vi "Vision_Processing_L_R1.vi"(0 "Current State":enum16{"Short Range", "Long Range"}(ring)=enum."Long Range", 1 "Image Dst":T1=refnum, 2 "Inpute Image":T1=refnum, 3 "Startup Flag":bool, 4 "Valid Beacon History - in":bool[](array[boolean])=[TRUE, TRUE, TRUE, TRUE, TRUE, TRUE, TRUE, TRUE, TRUE, TRUE, TRUE, TRUE, TRUE, TRUE, TRUE, TRUE, TRUE, TRUE, TRUE, TRUE], 5 "Current ROI Descriptor":T7={"Global Rectangle"=[0, 126, 320, 179], "Contours"=[{"ID"=enum."External", "Type"=12, "Coordinates"=[0, 126, 320, 179, 0]}]} {"Contours"."Type" items=["No Selection", "Point", "Line", "Rectangle", "Oval", "Polygon", "Freehand Region", "Annulus", "Unused2", "Unused3", "Broken Line", "Freehand Line", "Rotated Rectangle"]}, 6 "Avg Score - Last":dbl=882.2747192382812, 7 "error in (no error)":errorcluster, 8 "Current Settings":T4={"Curve Parameters"={"Extraction Mode"=1, "Edge Threshold"=150, "Edge Filter Size"=0, "Min Length"=25, "Row Search Step Size"=15, "Col Search Step Size"=15, "Max Endpoint Gap"=2, "Closed"=TRUE, "Subpixel"=TRUE}, "Match Mode"={"Rotation"=TRUE, "Scale"=TRUE, "Occlusion"=TRUE, "Reserved"=FALSE, "Reserved"=FALSE, "Reserved"=FALSE}, "Range Settings"=[{"Match Constraints"=0, "Min"=-5.0, "Max"=5.0}, {"Match Constraints"=1, "Min"=77.28628845214844, "Max"=87.28628845214844}, {"Match Constraints"=2, "Min"=0.0, "Max"=25.0}], "Number of Matches"=1, "Minimum Match Score"=782.2747, "SubPixel Accuracy"=TRUE, "Adv. Geometric Match Options 2"=[{"Setup Data Item"=20, "Item Value"=0.0}, {"Setup Data Item"=22, "Item Value"=1.0}]} {"Curve Parameters"."Extraction Mode" items=["Normal", "Uniform Regions"]; "Curve Parameters"."Edge Filter Size" items=["Fine", "Normal", "Contour Tracing"]; "Curve Parameters"."Max Endpoint Gap" min=0; "Curve Parameters"."Col Search Step Size" min=1 max=255 step=1; "Curve Parameters"."Row Search Step Size" min=1 max=255 step=1; "Curve Parameters"."Min Length" min=0; "Curve Parameters"."Edge Threshold" min=1 max=350 step=1; "Range Settings"."Max" format="%.2f"; "Range Settings"."Min" format="%.2f"; "Range Settings"."Match Constraints" items=["Rotation Angle (degrees)", "Scale Factor (%)", "Occlusion (%)"]; "Adv. Geometric Match Options 2"."Setup Data Item" items=["Curve Extraction Mode", "Curve Edge Threshold", "Curve Edge Filter Size", "Min Curve Length", "Curve Row Search Step Size", "Curve Col Search Step Size", "Curve Max Endpoint Gap", "Extract Closed Curves", "Enable Subpixel Curve Extraction", "Enable Correlation Score", "Enable Subpixel Accuracy", "Subpixel Iterations", "Subpixel Tolerance", "Initial Match List Length", "Enable Target Template Curve Score", "Min Match Separation Distance", "Min Match Separation Angle", "Min Match Separation Scale", "Max Match Overlap", "Enable Coarse Result", "Enable Calibration Support", "Enable Contrast Reversal", "Search Strategy", "Refinement Match Factor", "Subpixel Match Factor"]}, 9 "Sub Beacon Search Enable":bool[](array[boolean])=[FALSE, FALSE, FALSE, FALSE, FALSE], 13 "Avg Scale - Last":dbl=82.28628845214844, 14 "Valid Score History":dbl[](array[numeric])=[882.2267456054688, 879.6480102539062, 889.1240844726562, 884.991455078125, 875.38330078125, 881.3228759765625, 879.0923461914062, 884.8130493164062, 869.0428466796875, 879.3259887695312, 878.3837280273438, 878.5771484375, 878.74462890625, 883.9327392578125, 889.0577392578125, 886.224365234375, 888.1887817382812, 886.6435546875, 888.8932495117188, 880.26025390625] format="%#_13g", 15 "Valid Scale History":dbl[](array[numeric])=[86.3126220703125, 81.15679931640625, 81.2668228149414, 81.51744842529297, 81.17774963378906, 81.44428253173828, 81.47639465332031, 81.52884674072266, 81.38125610351562, 86.32369232177734, 81.46265411376953, 81.3922348022461, 81.34772491455078, 81.08159637451172, 81.33423614501953, 81.38683319091797, 81.22872924804688, 81.17185974121094, 81.34151458740234, 81.41799926757812] format="%#_13g", 16 "History Size":i32=20) -> (10 "Valid Scale History\nOut":dbl[](array[numeric])=[81.32903289794922, 86.3126220703125, 81.15679931640625, 81.2668228149414, 81.51744842529297, 81.17774963378906, 81.44428253173828, 81.47639465332031, 81.52884674072266, 81.38125610351562, 86.32369232177734, 81.46265411376953, 81.3922348022461, 81.34772491455078, 81.08159637451172, 81.33423614501953, 81.38683319091797, 81.22872924804688, 81.17185974121094, 81.34151458740234] format="%#_13g", 11 "Avg Scale":dbl=82.31654510498046, 12 "Avg Score":dbl=881.4775024414063, 17 "Valid Score History\nOut":dbl[](array[numeric])=[871.397216796875, 882.2267456054688, 879.6480102539062, 889.1240844726562, 884.991455078125, 875.38330078125, 881.3228759765625, 879.0923461914062, 884.8130493164062, 869.0428466796875, 879.3259887695312, 878.3837280273438, 878.5771484375, 878.74462890625, 883.9327392578125, 889.0577392578125, 886.224365234375, 888.1887817382812, 886.6435546875, 888.8932495117188] format="%#_13g", 18 "Valid Beacon History\nOut":bool[](array[boolean])=[TRUE, TRUE, TRUE, TRUE, TRUE, TRUE, TRUE, TRUE, TRUE, TRUE, TRUE, TRUE, TRUE, TRUE, TRUE, TRUE, TRUE, TRUE, TRUE, TRUE], 19 "Y Coordinates":sgl[](array[numeric])=[0.0, 0.0, 153.47913, 150.49385, 148.50107], 20 "Beacons Found":bool[](array[boolean])=[FALSE, FALSE, TRUE, TRUE, TRUE], 21 "X Coordinates":sgl[](array[numeric])=[0.0, 0.0, 161.30458, 216.11124, 265.1904], 22 "Next Main ROI Descriptor":T6={"Global Rectangle"=[0, 126, 320, 176], "Contours"=[{"ID"=enum."External", "Type"=12, "Coordinates"=[0, 126, 320, 176, 0]}]} {"Contours"."Type" items=["No Selection", "Point", "Line", "Rectangle", "Oval", "Polygon", "Freehand Region", "Annulus", "Unused2", "Unused3", "Broken Line", "Freehand Line", "Rotated Rectangle"]}, 23 "Lock Status":bool=TRUE, 24 "Startup Flag - out":bool, 25 "New Settings":T4={"Curve Parameters"={"Extraction Mode"=1, "Edge Threshold"=150, "Edge Filter Size"=0, "Min Length"=25, "Row Search Step Size"=15, "Col Search Step Size"=15, "Max Endpoint Gap"=2, "Closed"=TRUE, "Subpixel"=TRUE}, "Match Mode"={"Rotation"=TRUE, "Scale"=TRUE, "Occlusion"=TRUE, "Reserved"=FALSE, "Reserved"=FALSE, "Reserved"=FALSE}, "Range Settings"=[{"Match Constraints"=0, "Min"=-5.0, "Max"=5.0}, {"Match Constraints"=1, "Min"=77.31654510498046, "Max"=87.31654510498046}, {"Match Constraints"=2, "Min"=0.0, "Max"=25.0}], "Number of Matches"=1, "Minimum Match Score"=781.4775, "SubPixel Accuracy"=TRUE, "Adv. Geometric Match Options 2"=[{"Setup Data Item"=20, "Item Value"=0.0}, {"Setup Data Item"=22, "Item Value"=1.0}]} {"Curve Parameters"."Extraction Mode" items=["Normal", "Uniform Regions"]; "Curve Parameters"."Edge Filter Size" items=["Fine", "Normal", "Contour Tracing"]; "Curve Parameters"."Max Endpoint Gap" min=0; "Curve Parameters"."Col Search Step Size" min=1 max=255 step=1; "Curve Parameters"."Row Search Step Size" min=1 max=255 step=1; "Curve Parameters"."Min Length" min=0; "Curve Parameters"."Edge Threshold" min=1 max=350 step=1; "Range Settings"."Max" format="%.2f"; "Range Settings"."Min" format="%.2f"; "Range Settings"."Match Constraints" items=["Rotation Angle (degrees)", "Scale Factor (%)", "Occlusion (%)"]}, 26 "Next State":enum16{"Short Range", "Long Range"}(ring)=enum."Long Range", 27 "Right Image 2":T1(plugin-control))   [LabVIEW 2015]
uses:
  <vilib>/vision/Image Controls.llb/IMAQ Image.ctl
  <vilib>/vision/Pattern Matching.llb/IMAQ Curve Parameters.ctl
  <vilib>/vision/Pattern Matching.llb/IMAQ Match Range Setting.ctl
panel:
  in  "Scale Decay \nFactor":dbl=0.5
  in  "Scale Decay \nFactor":dbl=5.0
  in  "Valid Treshold\nfor Lock":i16=5
  in  "Indivudual Beacon \nCushion (pixels)":sgl=5.0
  out "New Min Score":dbl=781.4775024414063
  out "New Low Scale":dbl=77.31654510498046
  out "New high Scale":dbl=87.31654510498046
  in  "Absolute\nMinimum Score":dbl=700.0
  in  "Absolute\nMaximum Scale":dbl=300.0
  in  "Absolute\nMinimum Scale":dbl=10.0
  in  "Default No Lock\nSetting Values":T5={"Min Scale"=50.0, "Max Scale"=150.0, "Min Score"=800.0}
  in  "Score\nCushion":dbl=100.0
  in  "Scale \nCushion":dbl=5.0
  in  "LR to SR\nTransition Scale":sgl=90.0
  in  "SR to LR\nTransition Scale":sgl=90.0
  in  "Timeout \nThrehsold":i32=1000
  in  "Main ROI Decay\nper Fail (pixels)":i32=20
  in  "ROI_factor(Horiztonal) LR":sgl=5.0
  in  "ROI_factor(vertical) LR":sgl=2.5
  in  "ROI_factor(vertical) SR":sgl=2.7
  in  "ROI_factor(Horiztonal) SR":sgl=2.0
  out "Current  Score":sgl=871.3972
  out "Current  Scale":sgl=81.32903
  in  "Fail Count - In":i32
  in  "Sub Beacon Template File Path - ARRAY":path[](array[path])=[path "/home/lvuser/natinst/bin/BeaconTemplates/Sub1.png", path "/home/lvuser/natinst/bin/BeaconTemplates/Sub2.png", path "/home/lvuser/natinst/bin/BeaconTemplates/Sub3.png", path "/home/lvuser/natinst/bin/BeaconTemplates/Sub4.png", path "/home/lvuser/natinst/bin/BeaconTemplates/Sub5.png"]
  in  "Short Range Template FIle Path":path=path "/home/lvuser/natinst/bin/BeaconTemplates/SR_Main.png"
  in  "Long Range Main\nBeacon File Path":path=path "/home/lvuser/natinst/bin/BeaconTemplates/LR_Main.png"
  # "FILE PATHS"
  # "INPUTS"
  # "CONFIG"
  # "OUTPUTS"
  # "Range"
  # "Range"
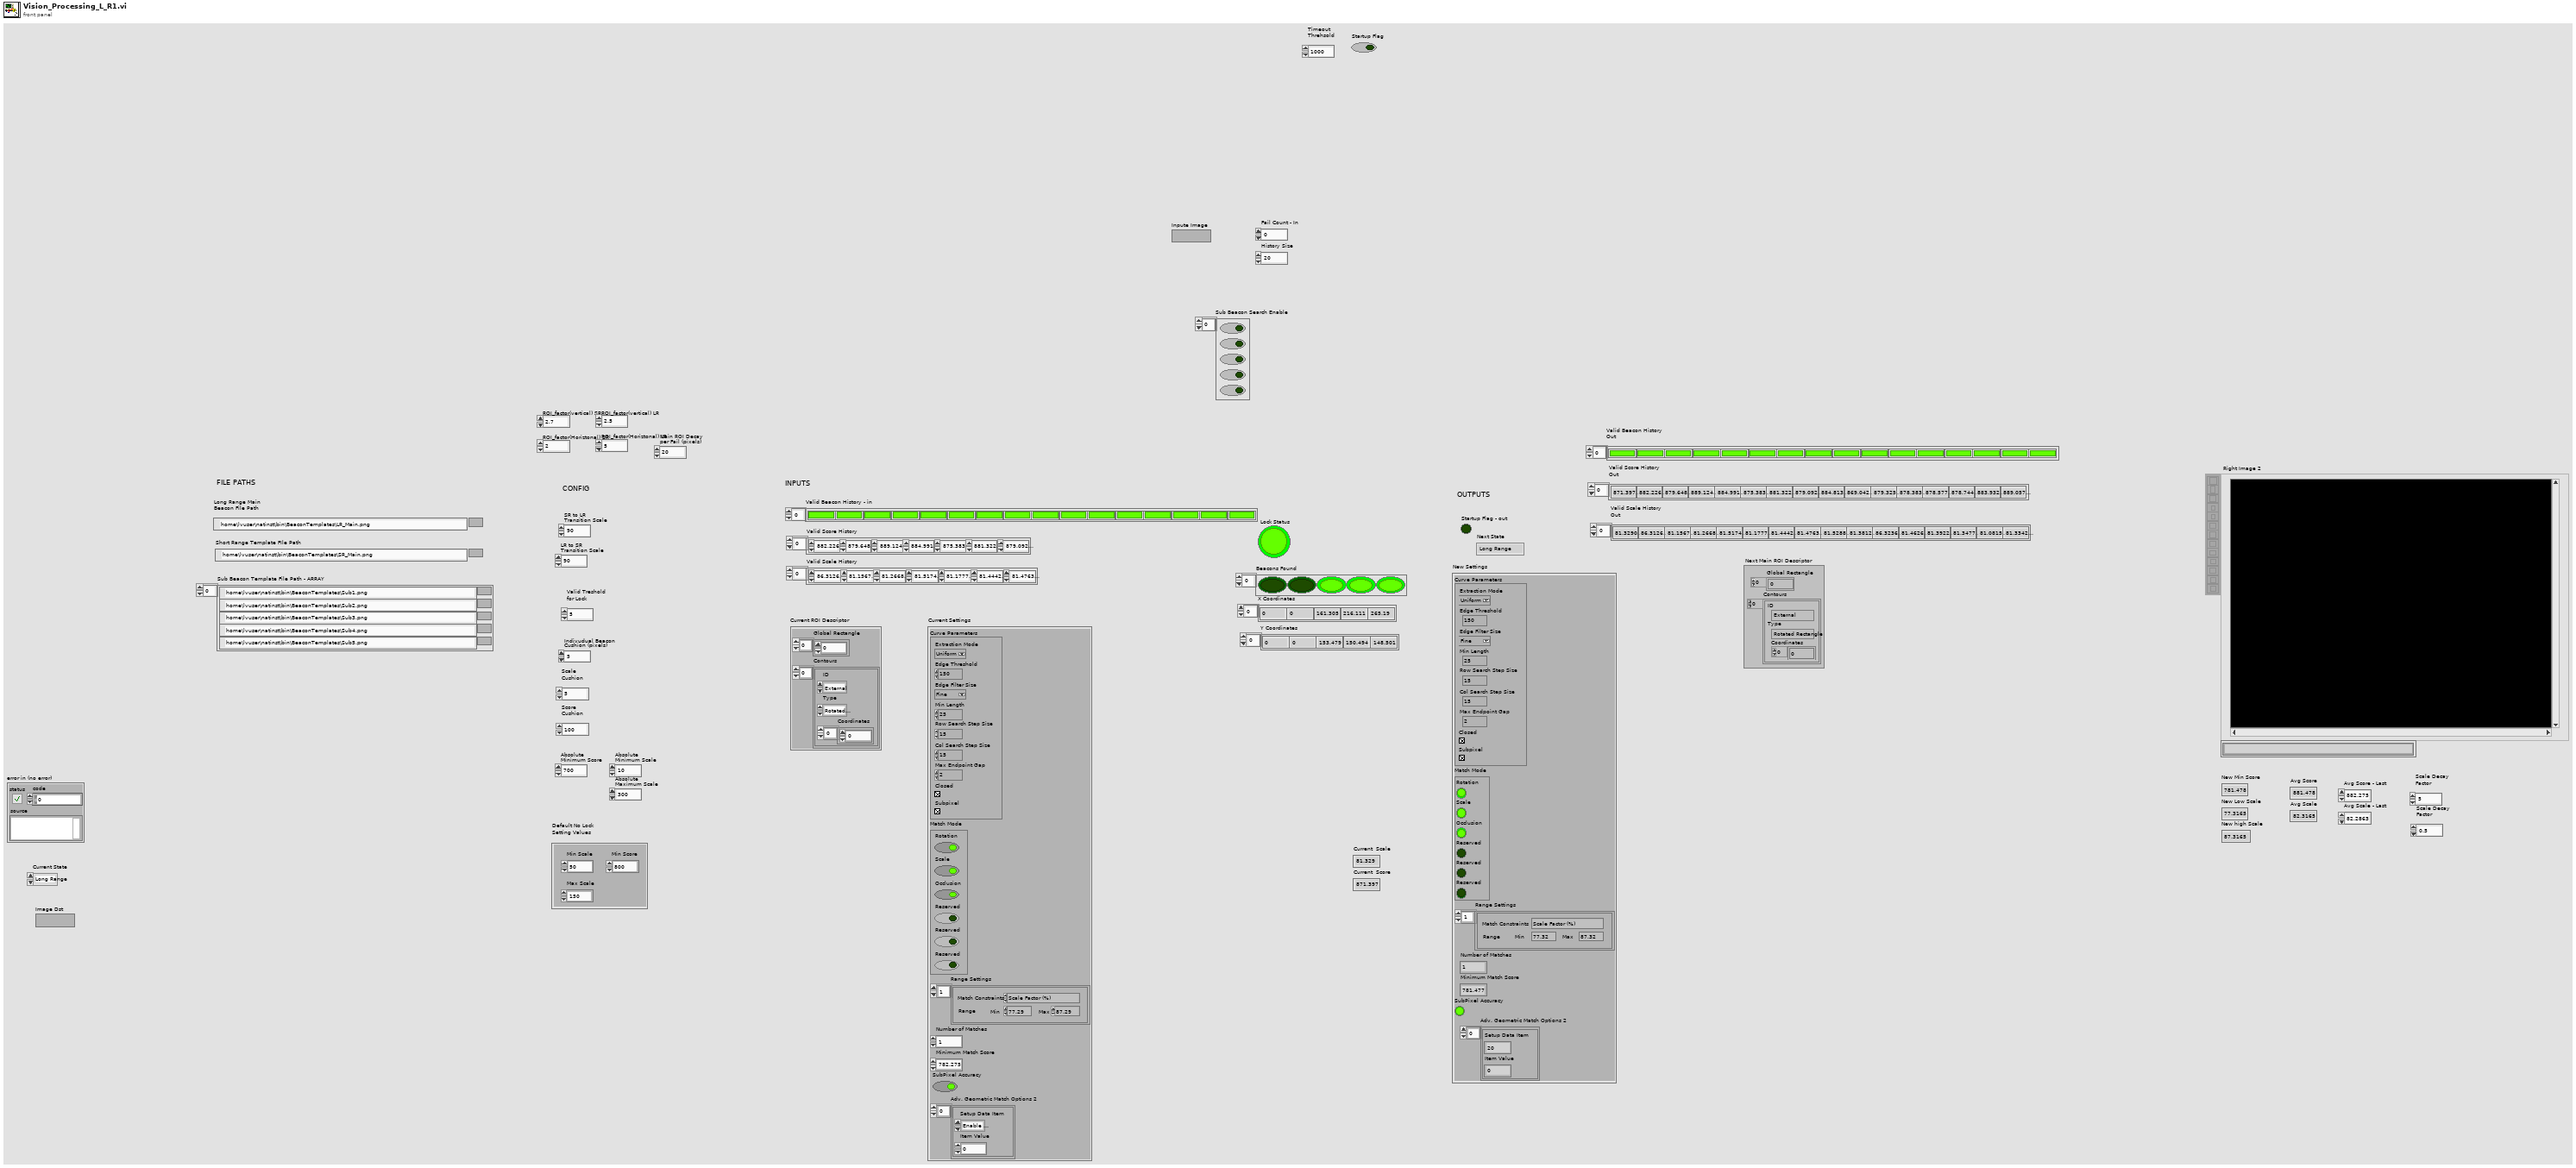
[diagram p1: front panel]
types:
  T1 = typedef "IMAQ Image.ctl" = refnum<image>
  T2 = typedef "IMAQ Curve Parameters.ctl" = cluster{"Extraction Mode":u32, "Edge Threshold":i32, "Edge Filter Size":u32, "Min Length":i32, "Row Search Step Size":i32, "Col Search Step Size":i32, "Max Endpoint Gap":i32, "Closed":bool, "Subpixel":bool}
  T3 = typedef "IMAQ Match Range Setting.ctl" = cluster{"Match Constraints":u32, "Min":dbl, "Max":dbl}
  T4 = cluster{"Curve Parameters":T2, "Match Mode":cluster{"Rotation":bool, "Scale":bool, "Occlusion":bool, "Reserved":bool, "Reserved":bool, "Reserved":bool}, "Range Settings":T3[], "Number of Matches":i32, "Minimum Match Score":sgl, "SubPixel Accuracy":bool, "Adv. Geometric Match Options 2":cluster{"Setup Data Item":u16, "Item Value":dbl}[]}
  T5 = cluster{"Min Scale":dbl, "Max Scale":dbl, "Min Score":dbl}
  T6 = typedef "ROI Descriptor" = cluster{"Global Rectangle":i32[], "Contours":cluster{"ID":enum32{"External", "Internal"}, "Type":u32, "Coordinates":i32[]}[]}
  T7 = cluster{"Global Rectangle":i32[], "Contours":cluster{"ID":enum32{"External", "Internal"}, "Type":u32, "Coordinates":i32[]}[]}
  T8 = typedef "IMAQ GM Match Report.ctl" = cluster{"Position":cluster{"x":sgl, "y":sgl}, "Angle":sgl, "Scale":sgl, "Score":sgl, "Bounding Box":cluster{"x":sgl, "y":sgl}[], "Contrast Reversed":bool, "Occlusion %":sgl, "Template Target Curve Score":sgl, "Target Template Curve Score":sgl, "Correlation Score":sgl}
  T9 = cluster{"Matches (Geometric Matching 1)[0]":T8, "Matches (Geometric Matching 1)[1]":T8, "Matches (Geometric Matching 1)[2]":T8, "Matches (Geometric Matching 1)[3]":T8, "Matches (Geometric Matching 1)[4]":T8, "Matches (Geometric Matching 1)[5]":T8, "Matches (Geometric Matching 1)[6]":T8, "Matches (Geometric Matching 1)[7]":T8, "Matches (Geometric Matching 1)[8]":T8}
  T10 = cluster{"Bounding Box[0]":cluster{"x":sgl, "y":sgl}, "Bounding Box[1]":cluster{"x":sgl, "y":sgl}, "Bounding Box[2]":cluster{"x":sgl, "y":sgl}, "Bounding Box[3]":cluster{"x":sgl, "y":sgl}, "Bounding Box[4]":cluster{"x":sgl, "y":sgl}, "Bounding Box[5]":cluster{"x":sgl, "y":sgl}, "Bounding Box[6]":cluster{"x":sgl, "y":sgl}, "Bounding Box[7]":cluster{"x":sgl, "y":sgl}, "Bounding Box[8]":cluster{"x":sgl, "y":sgl}}
  T11 = typedef "IMAQ Rectangle" = cluster{"Left":i32, "Top":i32, "Right":i32, "Bottom":i32, "Rotation":dbl}
  T12 = cluster{"index":u32, "Min Scale":dbl, "Max Scale":dbl}
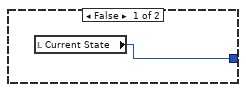
[diagram p2: hidden frame]
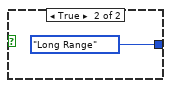
[diagram p3: hidden frame]
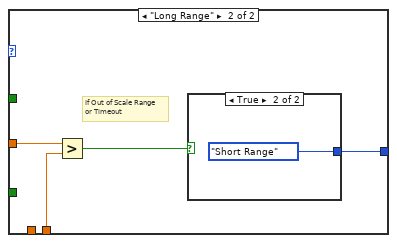
[diagram p4: hidden frame]
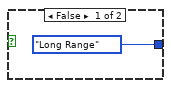
[diagram p5: hidden frame]
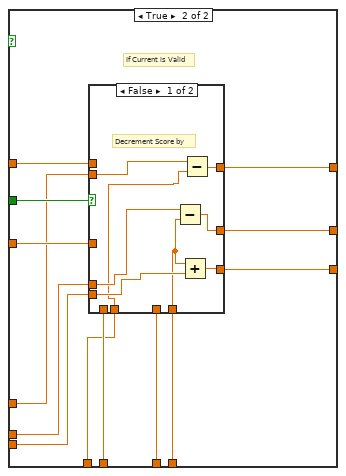
[diagram p8: hidden frame]
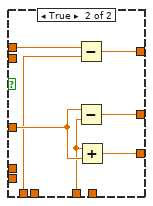
[diagram p9: hidden frame]
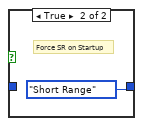
[diagram p10: hidden frame]
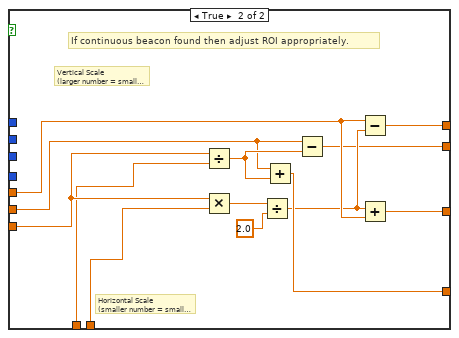
[diagram p12: hidden frame]
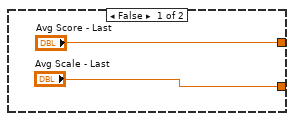
[diagram p13: hidden frame]
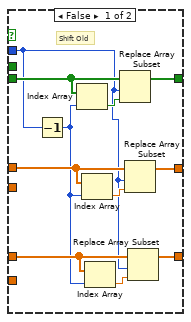
[diagram p15: hidden frame]
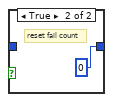
[diagram p16: hidden frame]
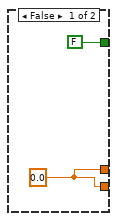
[diagram p17: hidden frame]
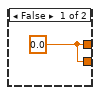
[diagram p18: hidden frame]
diagram:
  (unwired) enum16{"Short Range", "Long Range"}."Short Range"
  # "Next Settings"
  n1 = flat-sequence {
    tunnel: [w8] -> w3
    tunnel: [w7] -> w2
    tunnel: ["Image Dst"] -> w1
    tunnel: w3 -> [w135]
    tunnel: w2 -> [w133]
    tunnel: w1 -> [w134]
    frame #0 {
      # "APPLY FILTERING"
      n2 = call "Camera - Filtering"("Image In"="Inpute Image", "Image Dst"="Image Dst", "error in"="error in (no error)") -> ("Image Out"=w8:T1, "error out"=w7:errorcluster)  [unwired: 23 in]
    }
    frame #1 {
      w14 = 80.0 ("x")
      w48 = u32 1 ("index")
      w96 = u8 5
      # "Should be NEXT STATE"
      # "decay factor"
      # "Valid History"
      # "Draw ROI and stuff on outputi mage"
      # "Pull Down Startup IF Already True and Lock\nOtherwise don't update"
      # "Next Settings"
      # "Apply Limits to Settings"
      # "Scale"
      # "Min Score"
      # "Lower Scale"
      # "Upper Scale"
      # "Current Settings"
      # "Current Min\n& Max Scale"
      # "Current Valid"
      # "Update Search Settings"
      # "Next Template State"
      # "Update Template State"
      # "Calculate Average Scale/Score"
      # "Update Main ROI"
      # "Choose ROI Scale Factor"
      # "max avg"
      # "Min Required to use avarage"
      # "Valid  Ccount\n(up to 3)"
      # "****# of previous in history that must be true\nin order for position to be considered \"locked\""
      # "Update Shift Arrays"
      # "# of Beacons Found to be valid"
      # "Beacon - Y"
      # "Beacon - X"
      # "Beacons Found"
      # "Build ROI for Individual Beacons Based on Main Bounding Box"
      # "Starting X Lower Bound"
      # "Length of\nIndividual Beacon ROI"
      # "Length of Bounding Box"
      # "# of beacons"
      # "Outer Beacon Indexes"
      # "Matches"
      # "image out"
      n3 = case shown="False" "Startup Flag" {
        tunnel: [w200 enum16{"Short Range", "Long Range"}."Short Range"] -> w68
        tunnel: "Current State" -> [w200 _]
        frame False {
        }
        frame True {
          # "Force SR on Startup"
        }
      }
      n4 = case shown="\"Short Range\", Default" w68 {
        tunnel: w135 -> [w382 w417]
        tunnel: w134 -> [w381 w416]
        tunnel: "Current ROI Descriptor" -> [w379 w415]
        tunnel: "Current Settings" -> [w378 w414]
        tunnel: [1 0] -> w118
        tunnel: [3 4] -> w117
        tunnel: [w372 w408] -> w69
        tunnel: [w371 w407] -> w39
        tunnel: [w369 w405] -> w107
        tunnel: w133 -> [_ w404]
        tunnel: "Sub Beacon Search Enable" -> [w370 w403]
        tunnel: [sgl 3.0 ("y") sgl 5.0 ("y")] -> w119
        tunnel: [w367 w401] -> w115
        tunnel: [2 3] -> w108
        frame "Short Range", Default {
          n5 = call "Left Camera - Short Range"("Image In"=w382, "Image Dst"=w381, "ROI Descriptor (Geometric Matching 1)"=w379, "Settings (Geometric Matching 1)"=w378, "Template File Path (Geometric Matching 1)"="Short Range Template FIle Path") -> ("Image Out"=w371:T1, "Matches (Geometric Matching 1)"=w372:T8[], "Number of Matches (Geometric Matching 1)"=w373:i32, "error out"=w367:errorcluster)  [unwired: 19 in]
          n6 = Equal?(x=w373, y=1) -> (x = y?=w376:bool)
          n7 = case shown="True" w376 {
            tunnel: w370 -> [w390 w391]
            tunnel: [w383 w392] -> w369
            frame False {
              w384 = FALSE
              # "F"
              # "No Main Found,\nDon't Search any Subs"
              n8 = Replace Array Subset(array=w390, new element #1=w384, index #1=0 ("y"), new element #2=w384, index #2=1 ("y"), new element #3=w384, index #3=2 ("y"), new element #4=w384, index #4=3 ("y"), new element #5=w384, index #5=4 ("y")) -> (w383:bool[])
            }
            frame True {
              w393 = TRUE
              w394 = FALSE
              # "Search for MIDDLE Beacons"
              n9 = Replace Array Subset(array=w391, new element #1=w394, index #1=0 ("y"), new element #2=w393, index #2=1 ("y"), new element #3=w393, index #3=2 ("y"), new element #4=w393, index #4=3 ("y"), new element #5=w394, index #5=4 ("y")) -> (w392:bool[])
            }
          }
        }
        frame "Long Range" {
          n10 = call "Long Range"("Image In"=w417, "Image Dst"=w416, "ROI Descriptor (Geometric Matching 1)"=w415, "Settings (Geometric Matching 1)"=w414, "Template File Path (Geometric Matching 1)"="Long Range Main\nBeacon File Path", "error in"=w404) -> ("Image Out"=w407:T1, "Matches (Geometric Matching 1)"=w408:T8[], "Number of Matches (Geometric Matching 1)"=w410:i32, "error out"=w401:errorcluster)  [unwired: 18 in]
          n11 = Equal?(x=w410, y=1) -> (x = y?=w406:bool)
          n12 = case shown="True" w406 {
            tunnel: w403 -> [w425 w427]
            tunnel: [w418 w426] -> w405
            frame False {
              w419 = FALSE
              # "F"
              # "No Main Found,\nDon't Search any Subs"
              n13 = Replace Array Subset(array=w425, new element #1=w419, index #1=0 ("y"), new element #2=w419, index #2=1 ("y"), new element #3=w419, index #3=2 ("y"), new element #4=w419, index #4=3 ("y"), new element #5=w419, index #5=4 ("y")) -> (w418:bool[])
            }
            frame True {
              w428 = TRUE
              # "T"
              # "Search for ALL Beacons"
              n14 = Replace Array Subset(array=w427, new element #1=w428, index #1=0 ("y"), new element #2=w428, index #2=1 ("y"), new element #3=w428, index #3=2 ("y"), new element #4=w428, index #4=3 ("y"), new element #5=w428, index #5=4 ("y")) -> (w426:bool[])
            }
          }
        }
      }
      n15 = Array To Cluster(array=w69) -> (cluster=w131:T9)
      n16 = Unbundle By Name(w131) -> ("Matches (Geometric Matching 1)[0].Bounding Box"=w129:cluster{"x":sgl, "y":sgl}[], "Matches (Geometric Matching 1)[0].Scale"=w30:sgl, "Matches (Geometric Matching 1)[0].Score"=w29:sgl)
      "Current  Scale" <- w30
      "Current  Score" <- w29
      n17 = Array To Cluster(array=w129) -> (cluster=w130:T10)
      n18 = Unbundle By Name(w130) -> ("Bounding Box[0].x"=w123:sgl, "Bounding Box[0].y"=w122:sgl, "Bounding Box[2].x"=w121:sgl, "Bounding Box[2].y"=w120:sgl)
      n19 = Subtract(x=w121, y=w123) -> (x-y=w124:sgl)
      n20 = Divide(x=w124, y=w119) -> (x/y=w126:sgl)
      n21 = Subtract(x=w122, y="Indivudual Beacon \nCushion (pixels)") -> (x-y=w127:sgl)
      n22 = Add(x="Indivudual Beacon \nCushion (pixels)", y=w120) -> (x+y=w128:sgl)
      n23 = for {
        N: 5 -> [_]
        tunnel: w107 -> [w349] mode=indexing
        shift-right: [w332] -> _
        shift-left: w123 -> [w348]
        tunnel: w126 -> [w347]
        tunnel: w127 -> [w335]
        tunnel: w128 -> [w334]
        tunnel: [w333] -> w114 mode=indexing
        tunnel: w118 -> [w344]
        tunnel: w117 -> [w345]
        tunnel: "Indivudual Beacon \nCushion (pixels)" -> [w337]
        i -> [w346]
        # "Apply Horizontal Cushion to Outer Beacons"
        # "Divide Bounding Box"
        # "Upper Bound of Current is\nLower Bound for Next"
        n24 = case shown="True" w349 {
          tunnel: w348 -> [w362 w363]
          tunnel: w347 -> [_ w365]
          tunnel: [w362 w364] -> w338
          tunnel: [w362 w363] -> w341
          frame False {
            # "Don't Care"
          }
          frame True {
            # "X Lower Bound"
            n25 = Add(x=w363, y=w365) -> (x+y=w364:sgl)
          }
        }
        n26 = Equal?(x=w346, y=w344) -> (x = y?=w343:bool)
        n27 = case shown="True" w343 {
          tunnel: w341 -> [w357 w361]
          tunnel: [w357 w358] -> w340
          tunnel: [w356 w359] -> w339
          tunnel: w338 -> [w356 w359]
          tunnel: w337 -> [_ w360]
          frame False {
          }
          frame True {
            n28 = Subtract(x=w361, y=w360) -> (x-y=w358:sgl)
          }
        }
        n29 = Equal?(x=w346, y=w345) -> (x = y?=w342:bool)
        n30 = case shown="True" w342 {
          tunnel: w340 -> [w351 w355]
          tunnel: [w351 w354] -> w336
          tunnel: [w350 w352] -> w332
          tunnel: w339 -> [w350 w352]
          tunnel: w337 -> [_ w353]
          frame False {
          }
          frame True {
            n31 = Add(x=w355, y=w353) -> (x+y=w354:sgl)
          }
        }
        n32 = call "Bound_RO_R_R0I.vi"("Bottom Right - Y"=w334, "Right - X"=w332, "Top Left - Y"=w335, "Top  Left - x"=w336) -> ("ROI Descriptor"=w333:T6)  [unwired: 7 in]
      }
      n33 = for {
        N: 5 -> [_]
        tunnel: w39 -> [w313]
        tunnel: w115 -> [w312]
        tunnel: w114 -> [w311] mode=indexing
        tunnel: "Sub Beacon Template File Path - ARRAY" -> [w310] mode=indexing
        tunnel: [w309] -> w112 mode=indexing
        tunnel: [w308] -> w111 mode=indexing
        tunnel: [w307] -> w97 mode=indexing
        tunnel: w107 -> [w306] mode=indexing
        tunnel: "Current Settings" -> [w305]
        n34 = case shown="True" w306 {
          tunnel: w313 -> [_ w326]
          tunnel: w312 -> [_ w325]
          tunnel: w311 -> [_ w324]
          tunnel: w310 -> [_ w323]
          tunnel: [w314 w319] -> w309
          tunnel: [w314 w318] -> w308
          tunnel: [FALSE w317] -> w307
          tunnel: w305 -> [_ w316]
          frame False {
            w314 = sgl 0.0 ("x")
          }
          frame True {
            n35 = call "Sub Beacon Pattern Match"("Image In"=w326, "ROI Descriptor (Geometric Matching 1)"=w324, "Settings (Geometric Matching 1)"=w316, "Template File Path (Geometric Matching 1)"=w323, "error in"=w325) -> ("Matches (Geometric Matching 1)"=w320:T8[], "Number of Matches (Geometric Matching 1)"=w321:i32)  [unwired: 19 in, 2 out]
            n36 = Equal?(x=w321, y=1) -> (x = y?=w317:bool)
            n37 = case shown="True" w317 {
              tunnel: w320 -> [_ w330]
              tunnel: [w327 w329] -> w319
              tunnel: [w327 w328] -> w318
              frame False {
                w327 = sgl 0.0 ("x")
              }
              frame True {
                n38 = Array To Cluster(array=w330) -> (cluster=w331:T9)
                n39 = Unbundle By Name(w331) -> ("Matches (Geometric Matching 1)[0].Position.x"=w329:sgl, "Matches (Geometric Matching 1)[0].Position.y"=w328:sgl)
              }
            }
          }
        }
      }
      "Beacons Found" <- w97
      "X Coordinates" <- w112
      "Y Coordinates" <- w111
      n40 = local read "Current State"() -> (w70:enum16{"Short Range", "Long Range"})
      n41 = Boolean To (0,1)(Boolean=w97) -> (0, 1=w109:i16[])
      n42 = Add Array Elements(numeric array=w109) -> (sum=w110:i16)
      n43 = Array To Cluster(array=w69) -> (cluster=w73:T9)
      n44 = Greater Or Equal?(x=w110, y=w108) -> (x >= y?=w32:bool)
      n45 = Unbundle By Name(w73) -> ("Matches (Geometric Matching 1)[0].Position.x"=w78:sgl, "Matches (Geometric Matching 1)[0].Position.y"=w79:sgl, "Matches (Geometric Matching 1)[0].Scale"=w80:sgl)
      n46 = call "IMAQ Convert ROI to Rectangle"("ROI Descriptor"="Current ROI Descriptor") -> ("Rectangle"=w72:T11)  [unwired: 8 in, 1 out]
      n47 = case shown="False" w32 {
        tunnel: "Fail Count - In" -> [w303 _]
        tunnel: [w302 u16 0] -> w65
        frame False {
          n48 = Increment(x=w303) -> (x+1=w302:i32)
        }
        frame True {
          # "reset fail count"
        }
      }
      n49 = Unbundle By Name(w72) -> ("Left"=w74:i32, "Top"=w75:i32, "Right"=w76:i32, "Bottom"=w77:i32)
      n50 = Greater?(x=w65, y="Timeout \nThrehsold") -> (0:w64:bool)
      n51 = case shown="\"Long Range\"" w70 {
        tunnel: "ROI_factor(vertical) SR" -> [w203 _]
        tunnel: "ROI_factor(Horiztonal) SR" -> [w202 _]
        tunnel: "ROI_factor(vertical) LR" -> [_ w205]
        tunnel: "ROI_factor(Horiztonal) LR" -> [_ w204]
        tunnel: [w203 w205] -> w89
        tunnel: [w202 w204] -> w90
        frame "Short Range", Default {
        }
        frame "Long Range" {
        }
      }
      n52 = case shown="False" w32 {
        tunnel: w80 -> [_ w218]
        tunnel: w78 -> [_ w225]
        tunnel: w79 -> [_ w220]
        tunnel: [w210 w226] -> w84
        tunnel: [w209 w219] -> w81
        tunnel: [w208 w224] -> w82
        tunnel: [w207 w222] -> w83
        tunnel: w74 -> [w215 _]
        tunnel: w75 -> [w214 _]
        tunnel: w76 -> [w213 _]
        tunnel: w77 -> [w212 _]
        tunnel: w89 -> [_ w217]
        tunnel: w90 -> [_ w216]
        frame False {
          w206 = 3 ("y")
          n53 = Subtract(x=w215, y="Main ROI Decay\nper Fail (pixels)") -> (x-y=w210:i32)
          n54 = Subtract(x=w214, y=w206) -> (x-y=w209:i32)
          n55 = Add(x=w213, y="Main ROI Decay\nper Fail (pixels)") -> (x+y=w208:i32)
          n56 = Add(x=w212, y=w206) -> (x+y=w207:i32)
        }
        frame True {
          # "Horizontal Scale \n(smaller number = smaller ROI)"
          # "Vertical Scale \n(larger number = smaller ROI)"
          # "If continuous beacon found then adjust ROI appropriately."
          n57 = Divide(x=w218, y=w217) -> (x/y=w223:sgl)
          n58 = Multiply(x=w218, y=w216) -> (x*y=w228:sgl)
          n59 = Divide(x=w228, y=sgl 2.0) -> (x/y=w221:sgl)
          n60 = Add(x=w220, y=w223) -> (x+y=w222:sgl)
          n61 = Subtract(x=w220, y=w223) -> (x-y=w219:sgl)
          n62 = Subtract(x=w225, y=w221) -> (x-y=w226:sgl)
          n63 = Add(x=w225, y=w221) -> (x+y=w224:sgl)
        }
      }
      n64 = Decrement(x="History Size") -> (x-1=w105:i32)
      n65 = for {
        N: "History Size" -> [_]
        shift-right: [w280] -> w22
        shift-left: "Valid Beacon History - in" -> [w268]
        tunnel: w105 -> [w276]
        shift-right: [w273] -> w37
        shift-left: "Valid Score History" -> [w275]
        shift-right: [w272] -> w36
        shift-left: "Valid Scale History" -> [w274]
        tunnel: w29 -> [w271]
        tunnel: w30 -> [w270]
        tunnel: w32 -> [w269]
        i -> [w279]
        # "Reverse Index"
        n66 = Subtract(x=w276, y=w279) -> (x-y=w277:i32)
        n67 = Equal To 0?(x=w277) -> (x = 0?=w278:bool)
        n68 = case shown="True" w278 {
          tunnel: w277 -> [w281 w300]
          tunnel: w268 -> [w291 w293]
          tunnel: [w289 w292] -> w280
          tunnel: w269 -> [_ w301]
          tunnel: w275 -> [w286 w299]
          tunnel: w274 -> [w285 w298]
          tunnel: [w284 w296] -> w273
          tunnel: [w283 w297] -> w272
          tunnel: w271 -> [_ w295]
          tunnel: w270 -> [_ w294]
          frame False {
            # "Shift Old"
            n69 = Decrement(x=w281) -> (x-1=w282:i32)
            n70 = Index Array(array=w291, index=w282) -> (element=w290:bool)
            n71 = Index Array(array=w286, index=w282) -> (element=w288:dbl)
            n72 = Index Array(array=w285, index=w282) -> (element=w287:dbl)
            n73 = Replace Array Subset(array=w291, new element=w290, index=w281) -> (w289:bool[])
            n74 = Replace Array Subset(array=w286, new element=w288, index=w281) -> (w284:dbl[])
            n75 = Replace Array Subset(array=w285, new element=w287, index=w281) -> (w283:dbl[])
          }
          frame True {
            # "Scale"
            # "Score"
            # "Valid"
            # "insert New"
            n76 = Replace Array Subset(array=w299, new element=w295, index=w300) -> (w296:dbl[])
            n77 = Replace Array Subset(array=w298, new element=w294, index=w300) -> (w297:dbl[])
            n78 = Replace Array Subset(array=w293, new element=w301, index=w300) -> (w292:bool[])
          }
        }
      }
      "Valid Beacon History\nOut" <- w22
      "Valid Score History\nOut" <- w37
      "Valid Scale History\nOut" <- w36
      n79 = call "Bound_RO_R_R0I.vi"("Bottom Right - Y"=w83, "Right - X"=w82, "Top Left - Y"=w81, "Top  Left - x"=w84) -> ("ROI Descriptor"=w38:T6)  [unwired: 7 in]
      "Next Main ROI Descriptor" <- w38
      n80 = Boolean To (0,1)(Boolean=w22) -> (0, 1=w101:i16[])
      n81 = Add Array Elements(numeric array=w101) -> (sum=w102:i16)
      n82 = Greater Or Equal?(x=w102, y="Valid Treshold\nfor Lock") -> (x >= y?=w33:bool)
      "Lock Status" <- w33
      n83 = Initialize Array(u8 0, w96) -> (w99:u8[])
      n84 = while {
        shift-right: [w251] -> w94
        shift-left: w99 -> [w253]
        tunnel: w22 -> [w259] mode=indexing
        shift-right: [w257] -> w92
        shift-left: u8 0 -> [w260]
        tunnel: "History Size" -> [w258]
        tunnel: w96 -> [w250]
        i -> [w252]
        stop <- w254 stop-if-true
        # "Grab Last 2 Valid Indexes"
        n85 = case shown="True" w259 {
          tunnel: w260 -> [w262 w264]
          tunnel: [w262 w267] -> w257
          tunnel: w253 -> [w261 w266]
          tunnel: w252 -> [_ w265]
          tunnel: [w261 w263] -> w251
          frame False {
          }
          frame True {
            # "Update Index\nto use"
            # "Increment\nValid Count"
            n86 = Replace Array Subset(array=w266, new element=w265, index=w264) -> (w263:u8[])
            n87 = Increment(x=w264) -> (x+1=w267:u8)
          }
        }
        n88 = Greater?(x=w252, y=w258) -> (0:w255:bool)
        n89 = Greater Or Equal?(x=w257, y=w250) -> (x >= y?=w256:bool)
        n90 = Or(x=w256, y=w255) -> (x .or. y?=w254:bool)
      }
      n91 = Greater?(x=w92, y=u8 2) -> (0:w93:bool)
      n92 = case shown="True" w93 {
        tunnel: w92 -> [_ w234]
        tunnel: w94 -> [_ w240]
        tunnel: w37 -> [_ w239]
        tunnel: w36 -> [_ w238]
        tunnel: ["Avg Score - Last" w232] -> w26
        tunnel: ["Avg Scale - Last" w231] -> w27
        frame False {
        }
        frame True {
          w237 = 0.0
          n93 = for {
            N: w234 -> [_]
            tunnel: w240 -> [w247] mode=indexing
            tunnel: w239 -> [w249]
            tunnel: w238 -> [w248]
            shift-right: [w245] -> w236
            shift-left: w237 -> [w243]
            shift-right: [w246] -> w235
            shift-left: w237 -> [w242]
            # "Fetch Last Valid Values"
            n94 = Index Array(array=w249, index=w247) -> (element=w244:dbl)
            n95 = Index Array(array=w248, index=w247) -> (element=w241:dbl)
            n96 = Add(x=w244, y=w243) -> (x+y=w245:dbl)
            n97 = Add(x=w241, y=w242) -> (x+y=w246:dbl)
          }
          n98 = To Double Precision Float(number=w234) -> (double precision float=w233:dbl)
          n99 = Divide(x=w236, y=w233) -> (x/y=w232:dbl)
          n100 = Divide(x=w235, y=w233) -> (x/y=w231:dbl)
        }
      }
      "Avg Score" <- w26
      "Avg Scale" <- w27
      n101 = case shown="True" w33 {
        tunnel: w64 -> [_ w142]
        tunnel: "SR to LR\nTransition Scale" -> [_ w141]
        tunnel: "LR to SR\nTransition Scale" -> [_ w140]
        tunnel: w27 -> [_ w139]
        tunnel: w33 -> [_ w138]
        tunnel: [w136 w137] -> w34
        frame False {
          n102 = local read "Current State"() -> (w136:enum16{"Short Range", "Long Range"})
        }
        frame True {
          # "Timeout"
          # "Image Lock"
          n103 = local read "Current State"() -> (w143:enum16{"Short Range", "Long Range"})
          n104 = case shown="\"Short Range\", Default" w143 {
            tunnel: w138 -> [_ _]
            tunnel: w139 -> [w147 w152]
            tunnel: w142 -> [_ _]
            tunnel: w141 -> [w146 _]
            tunnel: w140 -> [_ w151]
            tunnel: [w144 w150] -> w137
            frame "Short Range", Default {
              # "If Out of Scale Range\nor Timeout"
              n105 = Less?(x=w147, y=w146) -> (x < y?=w145:bool)
              n106 = case shown="False" w145 {
                tunnel: [enum16{"Short Range", "Long Range"}."Short Range" ("Current State") enum16{"Short Range", "Long Range"}."Long Range" ("Current State")] -> w144
                frame False {
                }
                frame True {
                }
              }
            }
            frame "Long Range" {
              # "If Out of Scale Range\nor Timeout"
              n107 = Greater?(x=w152, y=w151) -> (0:w153:bool)
              n108 = case shown="True" w153 {
                tunnel: [enum16{"Short Range", "Long Range"}."Long Range" ("Current State") enum16{"Short Range", "Long Range"}."Short Range" ("Current State")] -> w150
                frame False {
                }
                frame True {
                }
              }
            }
          }
        }
      }
      "Next State" <- w34
      n109 = Unbundle By Name("Current Settings") -> ("Minimum Match Score"=w61:sgl, "Range Settings"=w45:T3[])
      n110 = Index Array(array=w45, index=u32 1) -> (element=w60:T3)
      n111 = Unbundle(w60) -> ("Min"=w58:dbl, "Max"=w57:dbl)  [unwired: 1 out]
      n112 = case shown="False" w33 {
        tunnel: w32 -> [_ w184]
        tunnel: w26 -> [w162 w183]
        tunnel: w27 -> [w161 w182]
        tunnel: w61 -> [_ w181]
        tunnel: w58 -> [_ w180]
        tunnel: w57 -> [_ w179]
        tunnel: [w160 w178] -> w46
        tunnel: [w159 w177] -> w10
        tunnel: [w158 w176] -> w12
        tunnel: "Scale \nCushion" -> [w164 w175]
        tunnel: "Score\nCushion" -> [w163 w174]
        tunnel: "Scale Decay \nFactor" -> [_ w173]
        tunnel: "Scale Decay \nFactor" -> [_ w172]
        frame False {
          # "Apply No Lock Default for each Template"
          n113 = Unbundle By Name("Default No Lock\nSetting Values") -> ("Min Score"=w160:dbl, "Min Scale"=w159:dbl, "Max Scale"=w158:dbl)
          n114 = disable-structure shown="Disabled" {
            disable-tunnel: [w171 _] -> _
            disable-tunnel: [w170 _] -> _
            disable-tunnel: w164 -> [w169 _]
            disable-tunnel: w163 -> [w168 _]
            disable-tunnel: w162 -> [w167 _]
            disable-tunnel: w161 -> [w166 _]
            frame Disabled {
              n115 = Subtract(x=w167, y=w168) -> ()  [unwired: 1 out]
              n116 = Subtract(x=w166, y=w169) -> (x-y=w171:dbl)
              n117 = Add(x=w169, y=w166) -> (x+y=w170:dbl)
            }
            frame Enabled {
            }
          }
        }
        frame True {
          # "If Current is Valid"
          n118 = case shown="False" w184 {
            tunnel: w183 -> [_ w199]
            tunnel: [w190 w198] -> w178
            tunnel: w182 -> [_ w197]
            tunnel: [w189 w196] -> w177
            tunnel: [w188 w195] -> w176
            tunnel: w180 -> [w192 _]
            tunnel: w179 -> [w191 _]
            tunnel: w181 -> [w187 _]
            tunnel: w175 -> [_ w194]
            tunnel: w174 -> [_ w193]
            tunnel: w173 -> [w186 _]
            tunnel: w172 -> [w185 _]
            frame False {
              # "Decrement Score by"
              n119 = Subtract(x=w192, y=w185) -> (x-y=w189:dbl)
              n120 = Add(x=w185, y=w191) -> (x+y=w188:dbl)
              n121 = Subtract(x=w187, y=w186) -> (x-y=w190:dbl)
            }
            frame True {
              n122 = Subtract(x=w199, y=w193) -> (x-y=w198:dbl)
              n123 = Subtract(x=w197, y=w194) -> (x-y=w196:dbl)
              n124 = Add(x=w194, y=w197) -> (x+y=w195:dbl)
            }
          }
        }
      }
      n125 = And(x="Startup Flag", y=w33) -> (x .and. y?=w42:bool)
      n126 = case shown="True" w42 {
        tunnel: "Startup Flag" -> [w156 _]
        tunnel: [w156 FALSE] -> w41
        frame False {
        }
        frame True {
        }
      }
      "Startup Flag - out" <- w41
      n127 = Subtract(x=w12, y=w14) -> (x-y=w16:dbl)
      n128 = Add(x=w14, y=w10) -> (x+y=w17:dbl)
      n129 = Less?(x=w12, y=w10) -> (x < y?=w19:bool)
      n130 = Greater?(x=w10, y=w12) -> (0:w18:bool)
      n131 = Select(t=w17, s=w19, f=w12) -> (s? t:f=w11:dbl)
      n132 = Select(t=w16, s=w18, f=w10) -> (s? t:f=w9:dbl)
      n133 = Less?(x=w46, y="Absolute\nMinimum Score") -> (x < y?=w50:bool)
      n134 = Less?(x=w9, y="Absolute\nMinimum Scale") -> (x < y?=w53:bool)
      n135 = Greater?(x=w11, y="Absolute\nMaximum Scale") -> (0:w55:bool)
      n136 = Select(t="Absolute\nMinimum Score", s=w50, f=w46) -> (s? t:f=w52:dbl)
      "New Min Score" <- w52
      n137 = Select(t="Absolute\nMinimum Scale", s=w53, f=w9) -> (s? t:f=w13:dbl)
      "New Low Scale" <- w13
      n138 = Select(t="Absolute\nMaximum Scale", s=w55, f=w11) -> (s? t:f=w15:dbl)
      "New high Scale" <- w15
      n139 = Bundle("index"=w48, "Min Scale"=w13, "Max Scale"=w15) -> (w47:T12)  [unwired: 1 in]
      n140 = Replace Array Subset(array=w45, new element=w47, index=w48) -> (w49:T3[])
      n141 = call "IMAQ Overlay ROI"("ROI Descriptor"=w38, "Image"=w39) -> ("Image Out"=→"Right Image 2":T1)  [unwired: 8 in, 1 out]
      n142 = Bundle By Name(cluster="Current Settings", "Range Settings"=w49, "Minimum Match Score"=w52) -> (→"New Settings":T4)
    }
  }
